vi "jimmy_stage_1.vi"() -> ()   [LabVIEW 2017]
panel:
  in  "Get position":bool
  out "Position status":dbl format="%.3f"
  in  "Target position":dbl format="%.3f"
  in  "Move":bool
  in  "Motor OFF":bool
  in  "Motor ON":bool
  in  "Step Size [um]":i32=10
  in  "Axis":i32=1
  in  "Rep Rate [Hz]":dbl=500.0
  out "Shots":dbl
  in  "Averaging Time [s]":dbl=0.1
  out "Current Point":i32
  out "Slide":i32(slide) scale=0.0..100.0
  out "Current Position [mm]":dbl
  in  "Axis initial position [mm]":dbl
  out "Axis final Position [mm]":dbl
  in  "Data Points (100 default)":i32=100
  in  "Collect Data!":bool
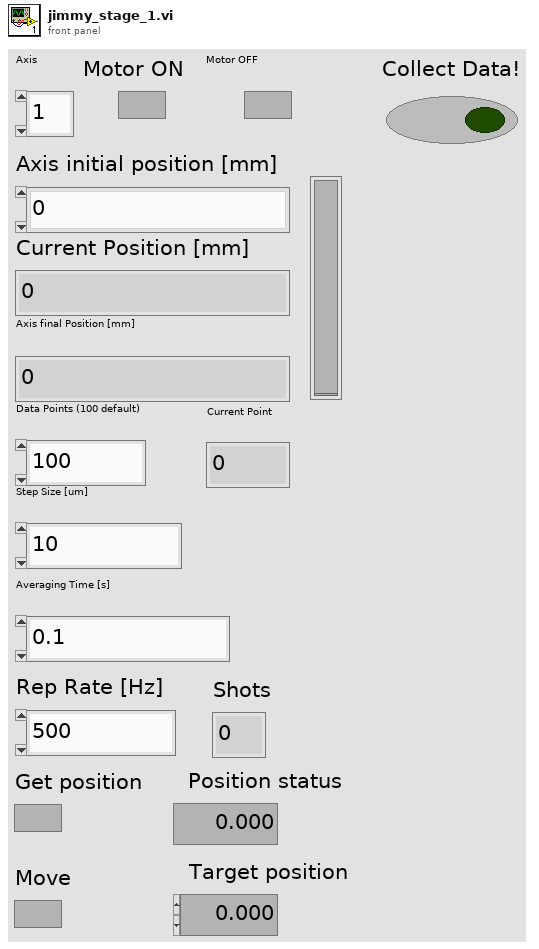
[diagram p1: front panel]
types:
  T1 = cluster{"input XON/XOFF":bool, "input HW Handshake":bool, "input alt HW HShk":bool, "output XON/XOFF":bool, "output HW Handshake":bool, "output alt HW HShk":bool, "XOFF byte":u8, "XON byte":u8, "parity error byte":u16}
  T2 = enum16{"no parity", "odd parity", "even parity", "mark parity", "space parity"}
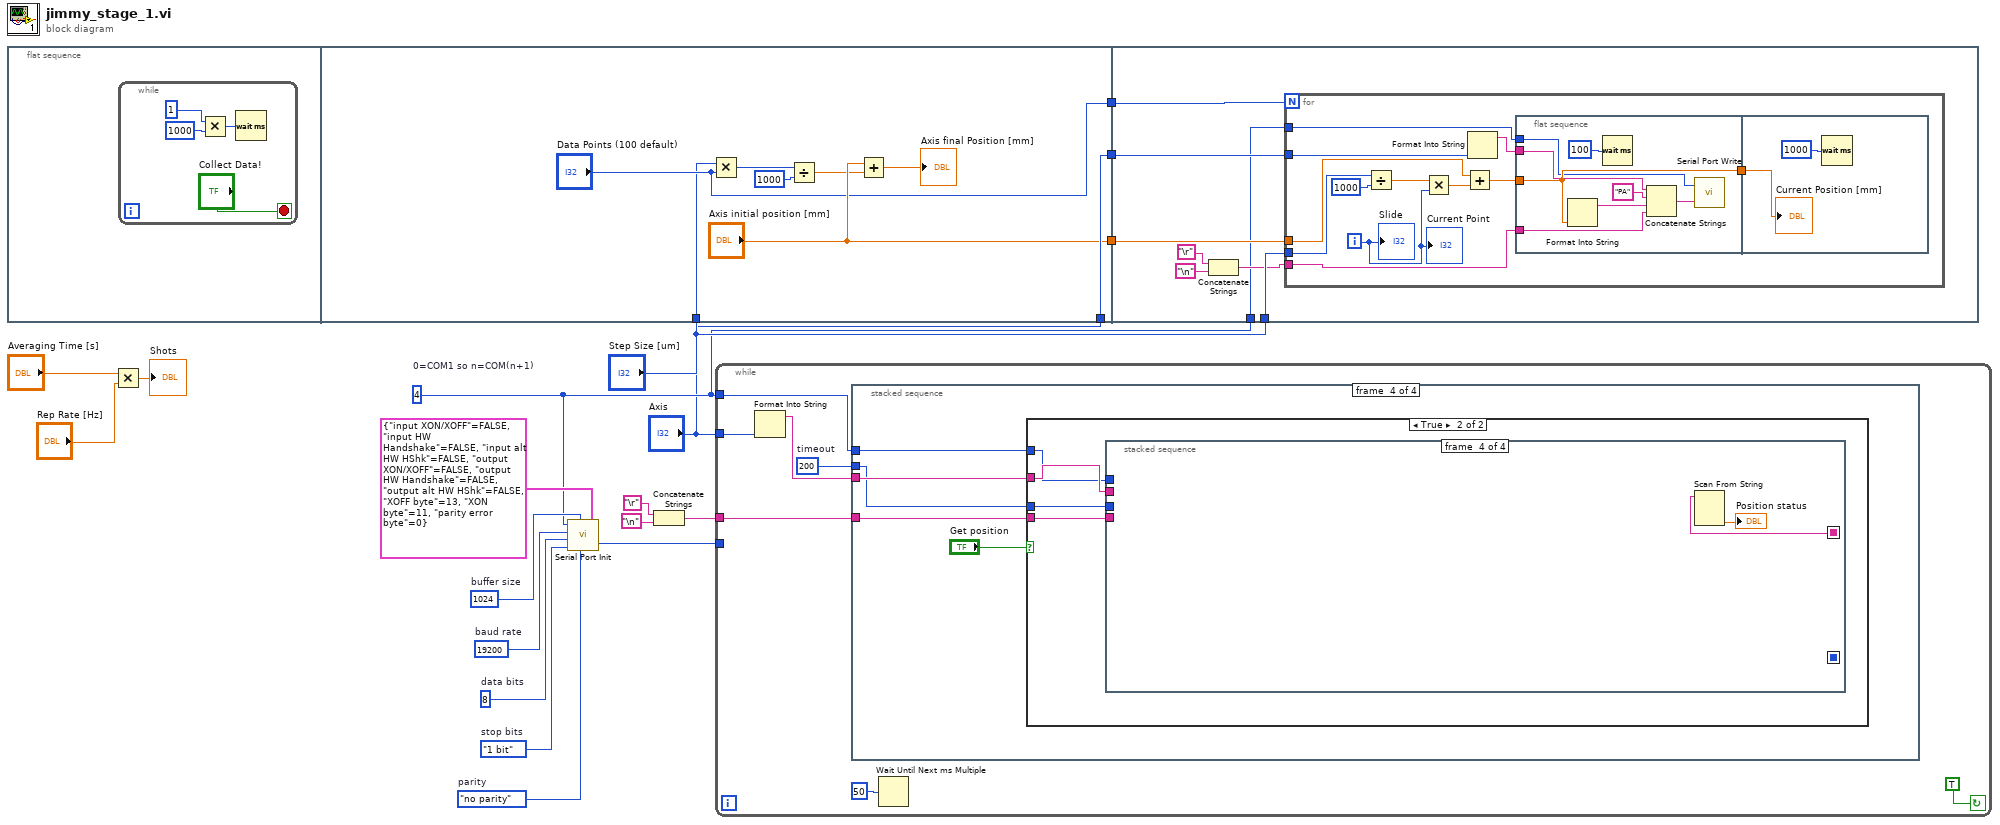
[diagram p0: block diagram]
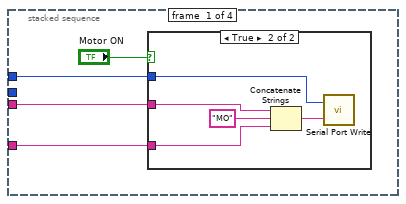
[diagram p2: hidden frame]
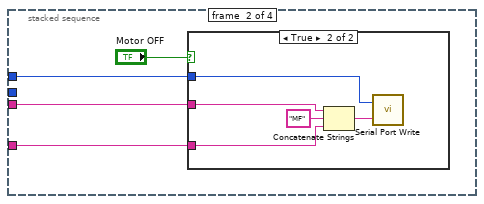
[diagram p4: hidden frame]
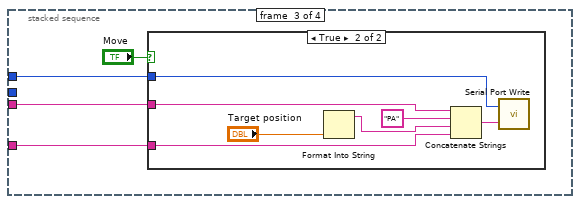
[diagram p6: hidden frame]
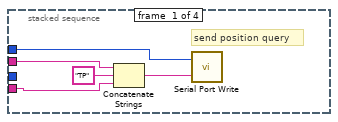
[diagram p9: hidden frame]
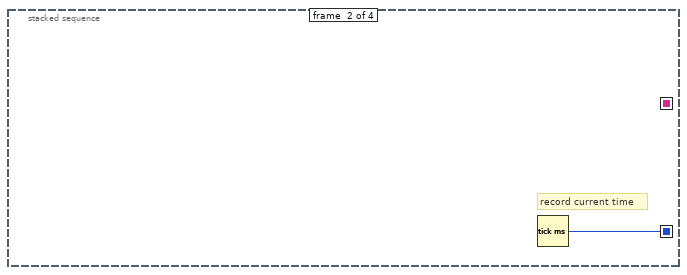
[diagram p10: hidden frame]
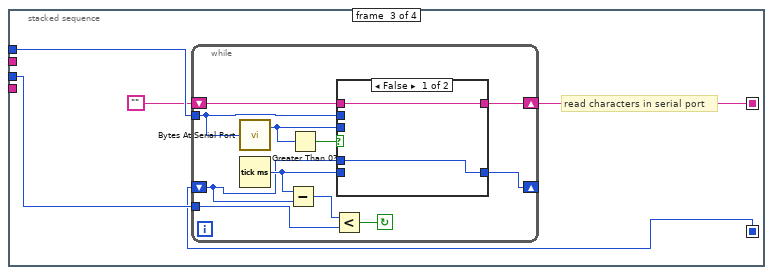
[diagram p11: hidden frame]
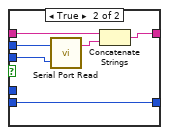
[diagram p12: hidden frame]
diagram:
  w9 = u32 19200  # baud rate
  w8 = u16 8  # data bits
  w7 = enum16{"1 bit", "1.5 bits", "2 bits"}."1 bit"  # stop bits
  w12 = T2."no parity"  # parity
  w6 = 4  # 0=COM1 so n=COM(n+1)
  w11 = u16 1024  # buffer size
  n1 = flat-sequence {
    tunnel: ["Data Points (100 default)"] -> w19
    tunnel: "Axis" -> [w31]
    tunnel: ["Axis initial position [mm]"] -> w18
    tunnel: "Step Size [um]" -> [w24]
    tunnel: [w31] -> w17
    tunnel: w19 -> [w39]
    tunnel: w18 -> [w38]
    tunnel: "Step Size [um]" -> [w37]
    tunnel: w17 -> [w36]
    tunnel: w6 -> [w32]
    frame #0 {
      n2 = while {
        stop <- "Collect Data!" stop-if-true
        n3 = Multiply(x=1, y=1000) -> (x*y=w23:i32)
        n4 = Wait (ms)(milliseconds to wait=w23) -> ()  [unwired: 1 out]
      }
    }
    frame #1 {
      n5 = Multiply(x=w24, y="Data Points (100 default)") -> (x*y=w27:i32)
      n6 = Divide(x=w27, y=1000) -> (x/y=w26:dbl)
      n7 = Add(x="Axis initial position [mm]", y=w26) -> (x+y=→"Axis final Position [mm]":dbl)
    }
    frame #2 {
      n8 = Concatenate Strings("\r", "\n") -> (w33:string)
      n9 = for {
        N: w39 -> [_]
        tunnel: w38 -> [w50]
        tunnel: w37 -> [w46]
        tunnel: w36 -> [w43]
        tunnel: w33 -> [w40]
        tunnel: w32 -> [w41]
        i -> [w51]
        n10 = Divide(x=w46, y=1000) -> (x/y=w45:dbl)
        n11 = Multiply(x=w45, y=w51) -> (x*y=w49:dbl)
        n12 = Add(x=w50, y=w49) -> (x+y=w48:dbl)
        n13 = Format Into String(w43) -> (resulting string=w42:string)  [unwired: 3 in, 1 out]
        n14 = flat-sequence {
          tunnel: w48 -> [w54]
          tunnel: [w54] -> w44
          tunnel: w40 -> [w56]
          tunnel: w42 -> [w55]
          tunnel: w41 -> [w52]
          tunnel: w44 -> [w60]
          frame #0 {
            n15 = Format Into String(w54) -> (resulting string=w53:string)  [unwired: 3 in, 1 out]
            n16 = Wait (ms)(milliseconds to wait=u32 100) -> ()  [unwired: 1 out]
            n17 = Concatenate Strings(w55, "PA" ("Substring"), w53, w56) -> (w58:string)
            n18 = call <vilib>:"Serial Port Write.vi"("string to write"=w58, "port number"=w52) -> ()  [unwired: 1 out]
          }
          frame #1 {
            n19 = Wait (ms)(milliseconds to wait=u32 1000) -> ()  [unwired: 1 out]
            "Current Position [mm]" <- w60
          }
        }
        "Current Point" <- w51
        "Slide" <- w51
      }
    }
  }
  n20 = Multiply(x="Averaging Time [s]", y="Rep Rate [Hz]") -> (x*y=→"Shots":dbl)
  n21 = call <vilib>:"Serial Port Init.vi"("flow control etc."=T1 {"input XON/XOFF"=FALSE, "input HW Handshake"=FALSE, "input alt HW HShk"=FALSE, "output XON/XOFF"=FALSE, "output HW Handshake"=FALSE, "output alt HW HShk"=FALSE, "XOFF byte"=13, "XON byte"=11, "parity error byte"=0}, "parity"=w12, "buffer size"=w11, "stop bits"=w7, "data bits"=w8, "baud rate"=w9, "port number"=w6) -> ("error code"=w5:i32)
  n22 = Concatenate Strings("\r", "\n") -> (w1:string)
  n23 = while {
    tunnel: w6 -> [w64]
    tunnel: w1 -> [w65]
    tunnel: w5 -> [_]
    tunnel: "Axis" -> [w62]
    stop <- TRUE continue-if-true
    w63 = u32 200  # timeout
    n24 = Format Into String(w62) -> (resulting string=w66:string)  [unwired: 3 in, 1 out]
    n25 = stacked-sequence {
      tunnel: w66 -> [w70 w80 w89 w101]
      tunnel: w65 -> [w69 w79 w88 w98]
      tunnel: w64 -> [w71 w81 w90 w100]
      tunnel: w63 -> [_ _ _ w99]
      frame #0 {
        n26 = case shown="True" "Motor ON" {
          tunnel: w71 -> [_ w77]
          tunnel: w70 -> [_ w74]
          tunnel: w69 -> [_ w73]
          frame False {
          }
          frame True {
            n27 = Concatenate Strings(w74, "MO" ("Substring"), w73) -> (w75:string)
            n28 = call <vilib>:"Serial Port Write.vi"("string to write"=w75, "port number"=w77) -> ()  [unwired: 1 out]
          }
        }
      }
      frame #1 {
        n29 = case shown="True" "Motor OFF" {
          tunnel: w81 -> [_ w86]
          tunnel: w80 -> [_ w83]
          tunnel: w79 -> [_ w82]
          frame False {
          }
          frame True {
            n30 = Concatenate Strings(w83, "MF" ("Substring"), w82) -> (w84:string)
            n31 = call <vilib>:"Serial Port Write.vi"("string to write"=w84, "port number"=w86) -> ()  [unwired: 1 out]
          }
        }
      }
      frame #2 {
        n32 = case shown="True" "Move" {
          tunnel: w90 -> [_ w97]
          tunnel: w89 -> [_ w94]
          tunnel: w88 -> [_ w93]
          frame False {
          }
          frame True {
            n33 = Format Into String("Target position") -> (resulting string=w91:string)  [unwired: 3 in, 1 out]
            n34 = Concatenate Strings(w94, "PA" ("Substring"), w91, w93) -> (w95:string)
            n35 = call <vilib>:"Serial Port Write.vi"("string to write"=w95, "port number"=w97) -> ()  [unwired: 1 out]
          }
        }
      }
      frame #3 {
        n36 = case shown="True" "Get position" {
          tunnel: w101 -> [_ w106]
          tunnel: w100 -> [_ w105]
          tunnel: w99 -> [_ w104]
          tunnel: w98 -> [_ w103]
          frame False {
          }
          frame True {
            n37 = stacked-sequence {
              seq-local: [_ w112 _ _] -> [_ _ w114 _]
              seq-local: [_ _ w113 _] -> [_ _ _ w138]
              tunnel: w106 -> [w109 _ _ _]
              tunnel: w105 -> [w108 _ w117 _]
              tunnel: w104 -> [_ _ w115 _]
              tunnel: w103 -> [w107 _ _ _]
              frame #0 {
                # "send position query"
                n38 = Concatenate Strings(w109, "TP" ("Substring"), w107) -> (w110:string)
                n39 = call <vilib>:"Serial Port Write.vi"("string to write"=w110, "port number"=w108) -> ()  [unwired: 1 out]
              }
              frame #1 {
                # "record current time"
                n40 = Tick Count (ms)() -> (millisecond timer value=w112:u32)
              }
              frame #2 {
                # "read characters in serial port"
                n41 = while {
                  shift-left: w114 -> [w118]
                  shift-right: [w119] -> _
                  tunnel: w115 -> [w122]
                  shift-left: "" -> [w125]
                  shift-right: [w124] -> w113
                  tunnel: w117 -> [w126]
                  stop <- w121 continue-if-true
                  n42 = call <vilib>:"Bytes At Serial Port.vi"("port number"=w126) -> ("byte count"=w127:u32)  [unwired: 1 out]
                  n43 = Tick Count (ms)() -> (millisecond timer value=w120:u32)
                  n44 = Subtract(x=w120, y=w118) -> (x-y=w123:u32)
                  n45 = Greater Than 0?(x=w127) -> (x > 0?=w128:bool)
                  n46 = Less?(x=w123, y=w122) -> (x < y?=w121:bool)
                  n47 = case shown="False" w128 {
                    tunnel: w127 -> [_ w136]
                    tunnel: w126 -> [_ w135]
                    tunnel: w125 -> [w130 w133]
                    tunnel: [w130 w132] -> w124
                    tunnel: [w129 w131] -> w119
                    tunnel: w120 -> [_ w131]
                    tunnel: w118 -> [w129 _]
                    frame False {
                    }
                    frame True {
                      n48 = call <vilib>:"Serial Port Read.vi"("requested byte count"=w136, "port number"=w135) -> ("string read"=w134:string)  [unwired: 1 out]
                      n49 = Concatenate Strings(w133, w134) -> (w132:string)
                    }
                  }
                }
              }
              frame #3 {
                n50 = Scan From String(input string=w138) -> (output 1=→"Position status":dbl)  [unwired: 4 in, 3 out]
              }
            }
          }
        }
      }
    }
    n51 = Wait Until Next ms Multiple(millisecond multiple=u32 50) -> ()  [unwired: 1 out]
  }
